vi "Stereo - Calibration Manager.vi"(7 "Function":T5, 10 "Right Grid Image":cluster{"Grid Image":T1, "Reference Points":T3}, 11 "Left Grid Image":cluster{"Grid Image":T1, "Reference Points":T3}) -> (0 "Calibration OK":bool, 1 "Calibrated Images":T1[](array[typedef]), 2 "Grid Coverage":T2, 3 "Grid Images out":cluster{"Left Image":T1, "Right Image":T1}[](array[cluster]))   [LabVIEW 2017]
doc: "Keeps track of the calibration grids needed to calibrate each camera.\nComputes the left and right camera models needed to compute the stereo calibration."
uses:
  Stereo - Calibration Manager Function.ctl
  <vilib>/vision/Image Controls.llb/IMAQ Image.ctl
  <vilib>/vision/Calibration.llb/Calibration Reference Points.ctl
  <vilib>/vision/Image Controls.llb/Vision Info Type2.ctl
  <vilib>/vision/NI_Vision_Development_Module.lvlib
panel:
  # "Overview: Keeps track of the calibration grids needed to calibrate each camera.\n                    Computes the left and right camera models needed to compute the stereo calibration."
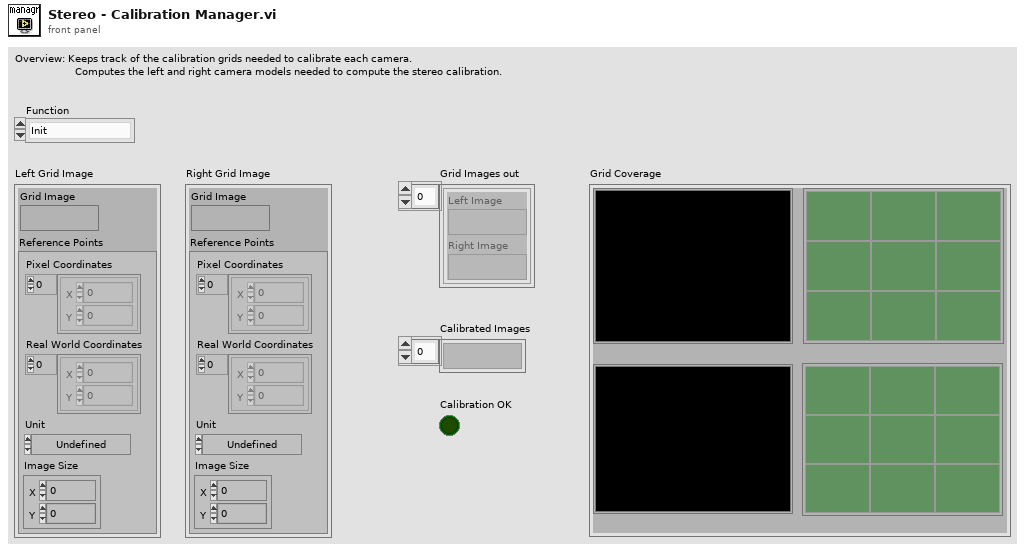
[diagram p1: front panel]
types:
  T1 = typedef "IMAQ Image.ctl" = refnum<image>
  T2 = cluster{"Left Image":T1, "Left Grid Coverage":bool[][], "Left Grid Coverage 3":string[][], "Right Image":T1, "Left Grid Coverage 2":bool[][], "Left Grid Coverage 4":string[][]}
  T3 = typedef "Calibration Reference Points.ctl" = cluster{"Pixel Coordinates":cluster{"X":dbl, "Y":dbl}[], "Real World Coordinates":cluster{"X":dbl, "Y":dbl}[], "Unit":T4, "Image Size":cluster{"X":u32, "Y":u32}}
  T4 = typedef "Image Unit" = enum32{"Undefined", "Angström", "Micrometer", "Millimeter", "Centimeter", "Meter", "Kilometer", "Microinch", "Inch", "Feet", "Nautical miles", "Standard miles", "Steps"}
  T5 = typedef "Stereo - Calibration Manager Function.ctl" = enum16{"Init", "Add Grid Images", "Get Images", "Dispose"}
  T6 = cluster{"Image Dst Out":T1, "Reference Points":T3}[][]
  T7 = cluster{"Left Image":T1, "Left Quadrants Status":bool[][], "Left Grid Coverage":string[][], "Right Image":T1, "Right Quadrant Status":bool[][], "Right Grid Coverage":string[][]}
  T8 = typedef "Vision Info Type2.ctl" = u32
  T9 = cluster{"Grid Image":T1, "Reference Points":T3}[]
  T10 = cluster{"Image Dst Out":T1, "Reference Points":T3}[]
  T11 = cluster{"Image Dst Out":T1, "Reference Points":T3}
  T12 = cluster{"Grid Image":T1, "Reference Points":T3}[][]
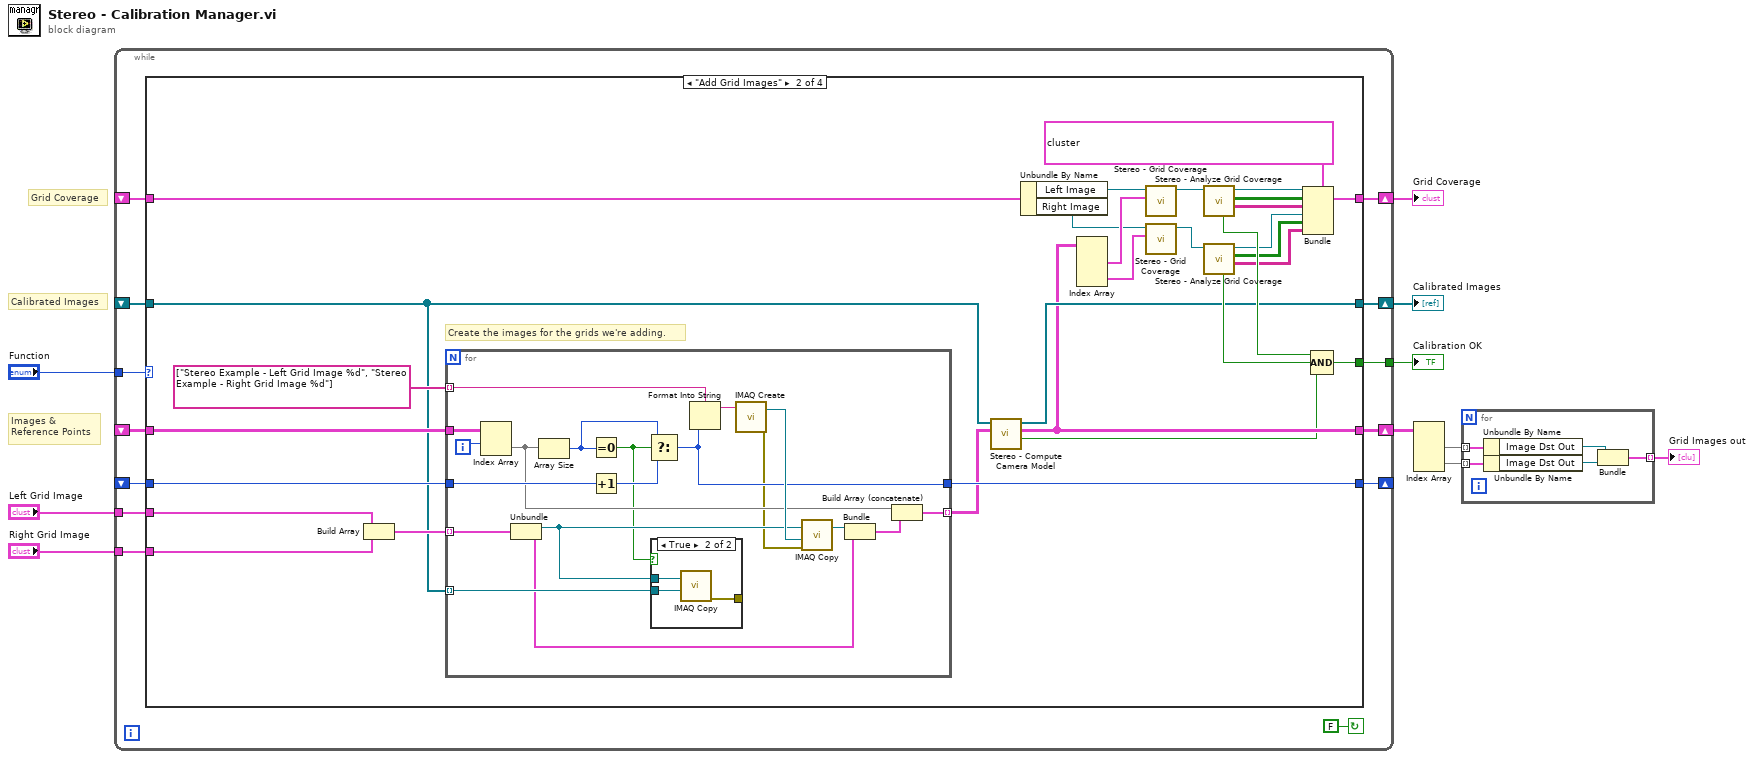
[diagram p0: block diagram]
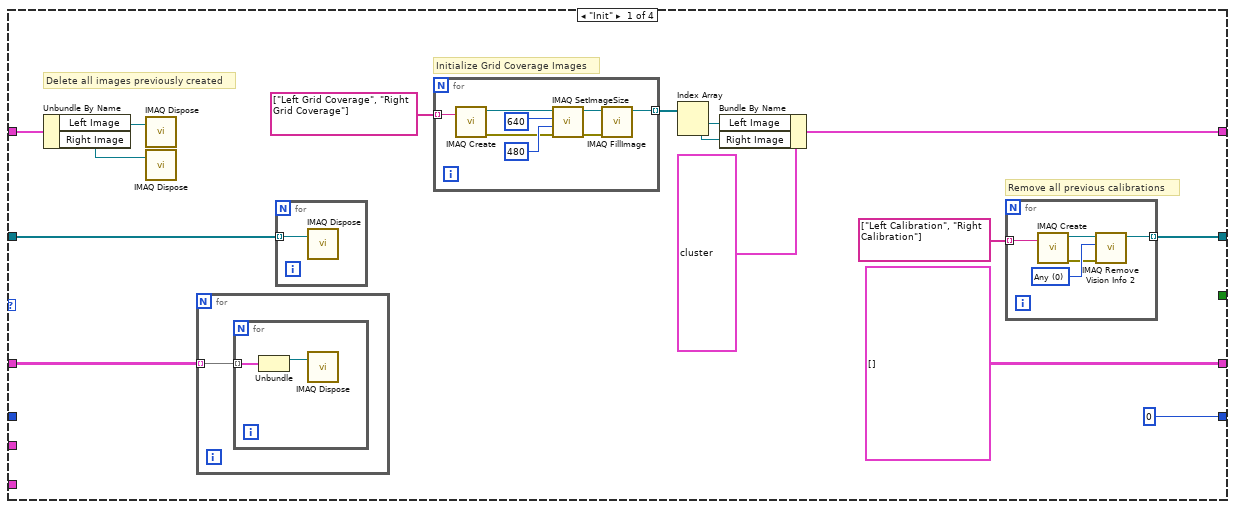
[diagram p2: hidden frame]
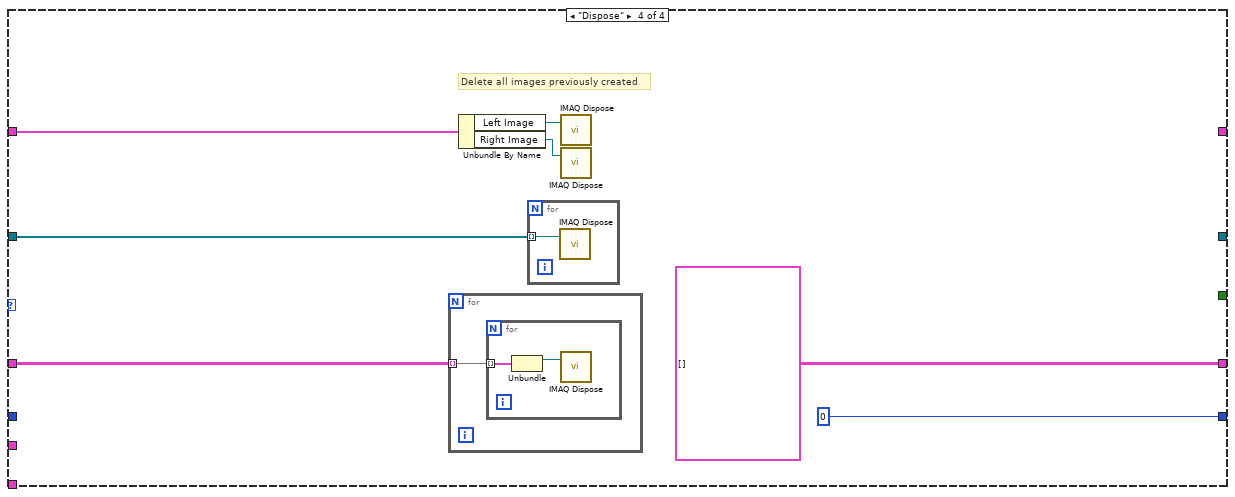
[diagram p5: hidden frame]
diagram:
  # "Calibrated Images"
  # "Grid Coverage"
  # "Images &\nReference Points"
  n1 = while {
    shift-right: [w23] -> w10
    shift-left: _ -> [w22]
    shift-right: [w19] -> w8
    shift-left: _ -> [w20]
    shift-right: [w17] -> _
    shift-left: _ -> [w18]
    shift-right: [w15] -> w5
    shift-left: _ -> [w16]
    tunnel: "Left Grid Image" -> [w14]
    tunnel: "Right Grid Image" -> [w13]
    tunnel: "Function" -> [w12]
    tunnel: [w11] -> w1
    stop <- FALSE continue-if-true
    n2 = case shown="\"Add Grid Images\"" w12 {
      tunnel: [w38 w58 w110 _] -> w23
      tunnel: w22 -> [w34 w60 w110 w115]
      tunnel: w20 -> [w37 w85 w111 w118]
      tunnel: [T6 [] w57 w111 T6 []] -> w19
      tunnel: w18 -> [_ w84 w109 _]
      tunnel: [0 w83 w109 0] -> w17
      tunnel: w16 -> [w33 w81 w108 w114]
      tunnel: [w32 w82 w108 _] -> w15
      tunnel: w14 -> [_ w80 _ _]
      tunnel: w13 -> [_ w79 _ _]
      tunnel: [_ w61 _ _] -> w11
      frame "Init" {
        # "Delete all images previously created"
        # "Remove all previous calibrations"
        # "Initialize Grid Coverage Images"
        n3 = Unbundle By Name(w33) -> ("Left Image"=w25:T1, "Right Image"=w24:T1)
        n4 = call "IMAQ Dispose"("Image"=w25) -> ()  [unwired: 2 in, 4 out]
        n5 = call "IMAQ Dispose"("Image"=w24) -> ()  [unwired: 2 in, 4 out]
        n6 = for {
          tunnel: w37 -> [w40] mode=indexing
          n7 = for {
            tunnel: w40 -> [w42] mode=indexing
            n8 = Unbundle(w42) -> ("Image Dst Out"=w41:T1)  [unwired: 1 out]
            n9 = call "IMAQ Dispose"("Image"=w41) -> ()  [unwired: 2 in, 4 out]
          }
        }
        n10 = for {
          tunnel: w34 -> [w39] mode=indexing
          n11 = call "IMAQ Dispose"("Image"=w39) -> ()  [unwired: 2 in, 4 out]
        }
        n12 = for {
          tunnel: string[] ["Left Grid Coverage", "Right Grid Coverage"] -> [w48] mode=indexing
          tunnel: [w47] -> w29 mode=indexing
          n13 = call "IMAQ Create"("Image Name"=w48) -> ("New Image"=w50:T1, "error out"=w43:errorcluster)  [unwired: 3 in, 1 out]
          n14 = call "IMAQ SetImageSize"("error in (no error)"=w43, "Y Resolution"=480 ("X Resolution"), "X Resolution"=640, "Image"=w50) -> ("error out"=w44:errorcluster, "Image Out"=w49:T1)  [unwired: 1 out]
          n15 = call "IMAQ FillImage"("error in (no error)"=w44, "Image"=w49) -> ("Image Out"=w47:T1)  [unwired: 5 in, 4 out]
        }
        n16 = Index Array(array=w29) -> (element #1=w27:T1, element #2=w26:T1)  [unwired: 2 in]
        n17 = Bundle By Name(cluster=T7 {"Left Image"=refnum, "Left Quadrants Status"=[], "Left Grid Coverage"=[], "Right Image"=refnum, "Right Quadrant Status"=[], "Right Grid Coverage"=[]} ("Grid Coverage 2"), "Left Image"=w27, "Right Image"=w26) -> (w32:T7)
        n18 = for {
          tunnel: string[] ["Left Calibration", "Right Calibration"] -> [w55] mode=indexing
          tunnel: [w52] -> w38 mode=indexing
          w53 = T8 0 items=["Any", "Calibration", "Overlay", "Grayscale Template", "Color Template", "Geometric Template", "Custom Data", "Golden Template", "Geometric Template 2", "Contour Data", "Camera Model"] ("Vision Info")
          n19 = call "IMAQ Create"("Image Name"=w55) -> ("New Image"=w54:T1, "error out"=w51:errorcluster)  [unwired: 3 in, 1 out]
          n20 = call "IMAQ Remove Vision Info 2"("error in (no error)"=w51, "Vision Info"=w53, "Image"=w54) -> ("Image Out"=w52:T1)  [unwired: 8 out]
        }
      }
      frame "Add Grid Images" {
        # "Create the images for the grids we're adding."
        n21 = Build Array(w80, w79) -> (w63:T9)
        n22 = for {
          tunnel: w84 -> [w100]
          tunnel: [w99] -> w83
          tunnel: w60 -> [w96] mode=indexing
          tunnel: w63 -> [w95] mode=indexing
          tunnel: string[] ["Stereo Example - Left Grid Image %d", "Stereo Example - Right Grid Image %d"] -> [w93] mode=indexing
          tunnel: w85 -> [w90]
          tunnel: [w88] -> w59 mode=indexing
          i -> [w89]
          n23 = Index Array(array=w90, index (row)=w89) -> (element=w91:T10)  [unwired: 1 in]
          n24 = Unbundle(w95) -> ("Grid Image"=w94:T1, "Reference Points"=w92:T3)
          n25 = Array Size(array=w91) -> (size(s)=w101:i32)
          n26 = Equal To 0?(x=w101) -> (x = 0?=w87:bool)
          n27 = Increment(x=w100) -> (x+1=w102:i32)
          n28 = Select(t=w101, s=w87, f=w102) -> (s? t:f=w99:i32)
          n29 = case shown="True" w87 {
            tunnel: w96 -> [_ w107]
            tunnel: w94 -> [_ w106]
            tunnel: [_ w105] -> _
            frame False {
            }
            frame True {
              n30 = call "IMAQ Copy"("Image Dst"=w107, "Image Src"=w106) -> ("error out"=w105:errorcluster)  [unwired: 1 in, 4 out]
            }
          }
          n31 = Format Into String(format string=w93, w99) -> (resulting string=w103:string)  [unwired: 2 in, 1 out]
          n32 = call "IMAQ Create"("Image Name"=w103) -> ("New Image"=w104:T1, "error out"=w86:errorcluster)  [unwired: 3 in, 1 out]
          n33 = call "IMAQ Copy"("error in (no error)"=w86, "Image Dst"=w104, "Image Src"=w94) -> ("Image Dst Out"=w98:T1)  [unwired: 4 out]
          n34 = Bundle("Image Dst Out"=w98, "Reference Points"=w92) -> (w97:T11)  [unwired: 1 out]
          n35 = Build Array (concatenate)(w91, w97) -> (w88:T10)
        }
        n36 = call "Stereo - Compute Camera Model.vi"("Images and Reference Points in"=w59, "Images"=w60) -> ("Boolean"=w56:bool, "Images and Reference Points out"=w57:T12, "Calibrated Images"=w58:T1[])  [unwired: 7 in]
        n37 = Unbundle By Name(w81) -> ("Left Image"=w70:T1, "Right Image"=w69:T1)
        n38 = Index Array(array=w57) -> (element #1=w78:T9, element #2=w77:T9)  [unwired: 4 in]
        n39 = call "Stereo - Grid Coverage.vi"("Grid Images"=w78, "Image in"=w70) -> ("Image out"=w76:T1)  [unwired: 1 in, 8 out]
        n40 = call "Stereo - Grid Coverage.vi"("Grid Images"=w77, "Image in"=w69) -> ("Image out"=w75:T1)  [unwired: 1 in, 8 out]
        n41 = call "Stereo - Analyze Grid Coverage.vi"("Grid Coverage"=w76) -> ("Coverage %"=w67:string[][], "Quadrants OK"=w68:bool[][], "Grid Coverage (dup)"=w74:T1, "Coverage OK"=w72:bool)  [unwired: 3 in, 4 out]
        n42 = call "Stereo - Analyze Grid Coverage.vi"("Grid Coverage"=w75) -> ("Coverage %"=w65:string[][], "Quadrants OK"=w66:bool[][], "Grid Coverage (dup)"=w71:T1, "Coverage OK"=w73:bool)  [unwired: 3 in, 4 out]
        n43 = Bundle(cluster=T7 {"Left Image"=refnum, "Left Quadrants Status"=[], "Left Grid Coverage"=[], "Right Image"=refnum, "Right Quadrant Status"=[], "Right Grid Coverage"=[]} ("Grid Coverage 2"), "Left Image"=w74, "Left Quadrants Status"=w68, "Left Grid Coverage"=w67, "Right Image"=w71, "Right Quadrant Status"=w66, "Right Grid Coverage"=w65) -> (w82:T7)
        n44 = Compound Arithmetic op=AND(w72, w73, w56) -> (w61:bool)
      }
      frame "Get Images" {
      }
      frame "Dispose" {
        # "Delete all images previously created"
        n45 = for {
          tunnel: w118 -> [w120] mode=indexing
          n46 = for {
            tunnel: w120 -> [w122] mode=indexing
            n47 = Unbundle(w122) -> ("Image Dst Out"=w121:T1)  [unwired: 1 out]
            n48 = call "IMAQ Dispose"("Image"=w121) -> ()  [unwired: 2 in, 4 out]
          }
        }
        n49 = Unbundle By Name(w114) -> ("Left Image"=w113:T1, "Right Image"=w112:T1)
        n50 = for {
          tunnel: w115 -> [w119] mode=indexing
          n51 = call "IMAQ Dispose"("Image"=w119) -> ()  [unwired: 2 in, 4 out]
        }
        n52 = call "IMAQ Dispose"("Image"=w113) -> ()  [unwired: 2 in, 4 out]
        n53 = call "IMAQ Dispose"("Image"=w112) -> ()  [unwired: 2 in, 4 out]
      }
    }
  }
  "Calibrated Images" <- w10
  "Grid Coverage" <- w5
  "Calibration OK" <- w1
  n54 = Index Array(array=w8) -> (element #1=w7:T10, element #2=w6:T10)  [unwired: 4 in]
  n55 = for {
    tunnel: [w125] -> w9 mode=indexing
    tunnel: w7 -> [w124] mode=indexing
    tunnel: w6 -> [w123] mode=indexing
    n56 = Unbundle By Name(w124) -> ("Image Dst Out"=w127:T1)
    n57 = Unbundle By Name(w123) -> ("Image Dst Out"=w126:T1)
    n58 = Bundle("Image Dst Out"=w127, "Image Dst Out"=w126) -> (w125:cluster{"Image Dst Out":T1, "Image Dst Out":T1})  [unwired: 1 out]
  }
  "Grid Images out" <- w9
